vi "main.vi"(8 "Error in":errorcluster) -> (0 "Error out":errorcluster)   [LabVIEW 2018, in "User Console.lvlib"]
uses:
  User Console.lvlib
  Common/Common.lvlib
  ctl/Module Queue - Action.ctl
  ctl/Module - State.ctl
  Common/ctl/Stop All - Action.ctl
  Error Handler/Error Handler.lvlib
  Error Handler/ctl/Module - State.ctl
  Controller/Controller.lvlib
  Controller/ctl/Module - State.ctl
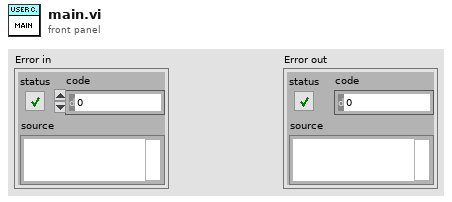
[diagram p1: front panel]
types:
  T1 = typedef "User Console.lvlib/Module Queue - Action.ctl" = enum16{"Create", "Get", "Destroy"}
  T2 = typedef "Common.lvlib/Stop All - Action.ctl" = enum16{"Create", "Fire", "Get", "Destroy"}
  T3 = typedef "User Console.lvlib/Module - State.ctl" = enum16{"Init", "Idle", "Error", "Close"}
  T4 = typedef "Controller.lvlib/Module - State.ctl" = enum16{"Init", "Idle", "Error", "Close"}
  T5 = typedef "Error Handler.lvlib/Module - State.ctl" = enum16{"Init", "Idle", "Error", "Close", "Handle External Error", "Log Error"}
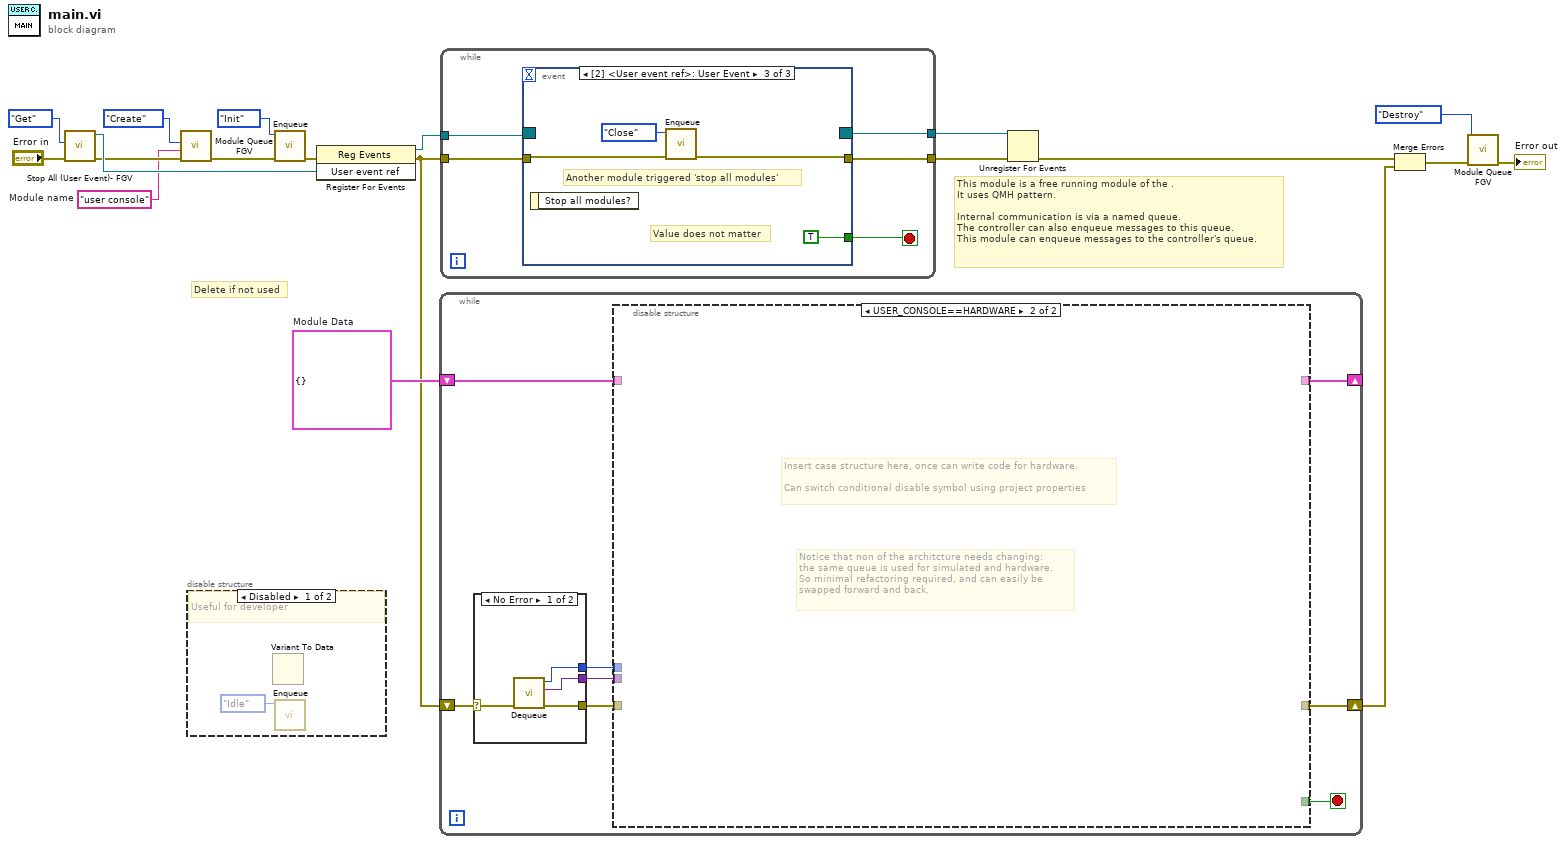
[diagram p0: block diagram]
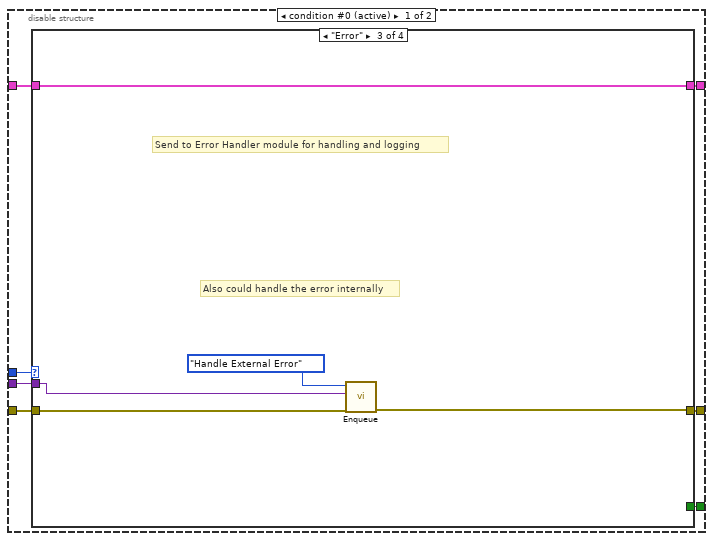
[diagram p2: hidden frame]
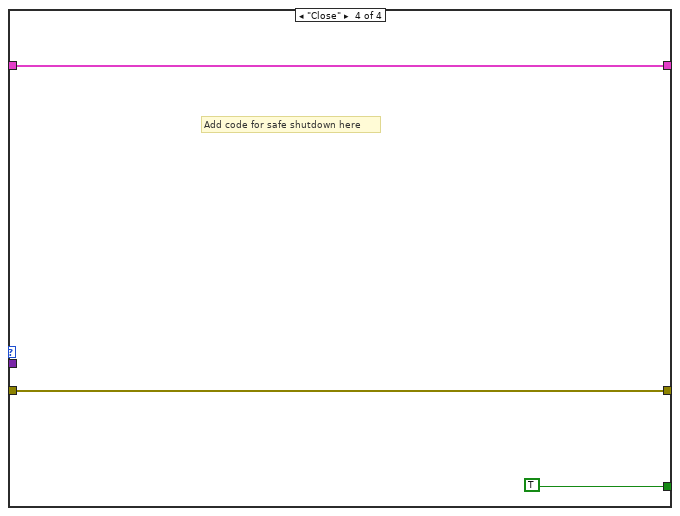
[diagram p5: hidden frame]
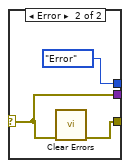
[diagram p6: hidden frame]
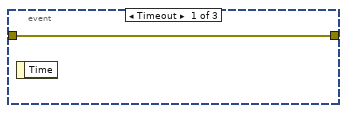
[diagram p8: hidden frame]
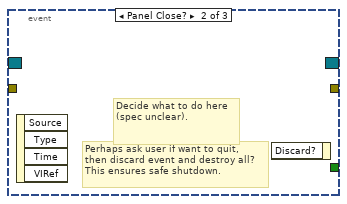
[diagram p9: hidden frame]
diagram:
  w1 = "user console"  # Module name
  w8 = cluster{} {}  # Module Data
  # "This module is a free running module of the .\nIt uses QMH pattern.\n\nInternal communication is via a named queue.\nThe controller can also enqueue messages to this queue.\nThis module can enqueue messages to the controller's queue."
  # "Delete if not used"
  n1 = call "Stop All (User Event)- FGV.vi"("error in"="Error in", "Action"=Stop_All_-_Action."Get") -> ("error out"=w10:errorcluster, "User event ref"=w15:refnum<user-event>)  [unwired: 8 in]
  n2 = call "Module Queue FGV.vi"("Error in"=w10, "Queue name"=w1, "Action"=Module_Queue_-_Action."Create") -> ("Error out"=w18:errorcluster)  [unwired: 7 in, 1 out]
  n3 = disable-structure shown="Disabled" {
    frame Disabled {
      # "Useful for developer"
      n4 = Variant To Data() -> ()  [unwired: 3 in, 2 out]
      n5 = call "Enqueue.vi"("State"=Module_-_State."Idle") -> ()  [unwired: 10 in, 1 out]
    }
    frame Enabled {
    }
  }
  n6 = call "Enqueue.vi"("error in (no error)"=w18, "State"=Module_-_State."Init") -> ("error out"=w9:errorcluster)  [unwired: 9 in]
  n7 = register-events(error in=w9, w15) -> (reference out=w13:refnum<event-registration>, error out=w3:errorcluster)  [unwired: 1 in]
  n8 = while {
    shift-right: [w28] -> _
    shift-left: w8 -> [w27]
    shift-right: [w21] -> w2
    shift-left: w3 -> [w26]
    stop <- w22 stop-if-true
    n9 = case shown="No Error" w26 {
      selector: w26 -> [w50 w52]
      tunnel: [w49 Module_-_State."Error" ("State")] -> w25
      tunnel: [w48 w52] -> w24
      tunnel: [w47 w51] -> w23
      frame No Error {
        n10 = call "Dequeue.vi"("error in"=w50) -> ("error out"=w47:errorcluster, "Data"=w48:variant, "State"=w49:T3)  [unwired: 8 in]
      }
      frame Error {
        # "Instead of dequeue,\nhandle the error"
        n11 = call <vilib>:"Clear Errors.vi"("error in (no error)"=w52) -> ("error out"=w51:errorcluster)  [unwired: 5 in, 1 out]
      }
    }
    n12 = disable-structure shown="USER_CONSOLE==HARDWARE" {
      disable-tunnel: [w35 _] -> w28
      disable-tunnel: w27 -> [w34 _]
      disable-tunnel: w25 -> [w33 _]
      disable-tunnel: w24 -> [w32 _]
      disable-tunnel: w23 -> [w31 _]
      disable-tunnel: [w30 _] -> w22
      disable-tunnel: [w29 _] -> w21
      frame condition #0 (active) {
        n13 = case shown="\"Error\"" w33 {
          tunnel: [w36 w38 w43 w44] -> w35
          tunnel: w34 -> [w36 w38 w43 w44]
          tunnel: w32 -> [_ _ w40 _]
          tunnel: w31 -> [_ w37 w42 w45]
          tunnel: [_ _ _ TRUE] -> w30
          tunnel: [_ w37 w41 w45] -> w29
          frame "Init", Default {
          }
          frame "Idle" {
          }
          frame "Error" {
            # "Send to Error Handler module for handling and logging"
            # "Also could handle the error internally"
            n14 = call "Enqueue.vi"("error in (no error)"=w42, "Data"=w40, "State"=Module_-_State."Handle External Error") -> ("error out"=w41:errorcluster)  [unwired: 8 in]
          }
          frame "Close" {
            # "Add code for safe shutdown here"
          }
        }
      }
      frame condition #1 {
        # "Notice that non of the architcture needs changing:\nthe same queue is used for simulated and hardware.\nSo minimal refactoring required, and can easily be \nswapped forward and back."
        # "Insert case structure here, once can write code for hardware.\n\nCan switch conditional disable symbol using project properties"
      }
    }
  }
  n15 = while {
    tunnel: w13 -> [w58]
    tunnel: [w57] -> w12
    tunnel: w3 -> [w56]
    tunnel: [w55] -> w11
    stop <- w54 stop-if-true
    n16 = event shown="[2] <User event ref>: User Event" {
      selector: w58 -> [_ _ _]
      dyn-events: [_ _ _] -> w57
      timeout: _ -> [_ _ _]
      tunnel: w56 -> [w59 _ w63]
      tunnel: [w59 _ w62] -> w55
      tunnel: [_ _ TRUE] -> w54
      event Timeout {
        n17 = event-data() -> ()  [unwired: 1 in, 1 out]
      }
      event Panel Close? {
        # "Perhaps ask user if want to quit,\nthen discard event and destroy all?\nThis ensures safe shutdown."
        # "Decide what to do here\n(spec unclear)."
        n18 = event-data() -> ()  [unwired: 1 in, 4 out]
        n19 = event-data() -> ()  [unwired: 2 in, 1 out]
      }
      event User Event {
        # "Value does not matter"
        # "Another module triggered 'stop all modules'"
        n20 = event-data() -> ()  [unwired: 1 in, 1 out]
        n21 = call "Enqueue.vi"("error in (no error)"=w63, "State"=Module_-_State."Close") -> ("error out"=w62:errorcluster)  [unwired: 9 in]
      }
    }
  }
  n22 = Unregister For Events(event registration refnum=w12, error in=w11) -> (error out=w7:errorcluster)
  n23 = Merge Errors(w7, w2) -> (w6:errorcluster)
  n24 = call "Module Queue FGV.vi"("Error in"=w6, "Action"=Module_Queue_-_Action."Destroy") -> ("Error out"=→"Error out":errorcluster)  [unwired: 8 in, 1 out]
